vi "svx_Shortcut Menu.vi"(7 "waveform graph?":bool, 9 "Container State":T3, 10 "Display State In":T1={"X Scale Width %"=50.0, "Y Scale Height %"=50.0, "X-Axis Range"={"Minimum"=0.0, "Maximum"=10.0}, "Y-Axis Range"={"Minimum"=0.0, "Maximum"=10.0}, "Z-Axis Range"={"Minimum"=0.0, "Maximum"=10.0}, "Plot Color"=61212, "Frame Color"=16252785, "Background Color"=16777222, "Initial AutoScale Y"=TRUE, "AutoScale X"=2, "AutoScale Y"=2, "AutoScale Z"=2, "Plot Transparency"=FALSE, "X-Axis Name"="Frequency", "Y-Axis Name"="Amplitude", "Z-Axis Name"="", "X-Axis Scaling Factor"={"Offset"=0.0, "Multiplier"=1.0}, "Y-Axis Scaling Factor"={"Offset"=0.0, "Multiplier"=1.0}, "Z-Axis Scaling Factor"={"Offset"=0.0, "Multiplier"=1.0}, "X-Scale Visible"=TRUE, "Y-Scale Visible"=TRUE, "Z-Scale Visible"=TRUE, "X-Scale Label Visible"=TRUE, "Y-Scale Label Visible"=TRUE, "Z-Scale Label Visible"=TRUE, "X-Axis Range Scaled"={"Minimum"=0.0, "Maximum"=10.0}, "Y-Axis Range Scaled"={"Minimum"=0.0, "Maximum"=10.0}, "Z-Axis Range Scaled"={"Minimum"=0.0, "Maximum"=10.0}, "Rev Z Order"=FALSE, "X-Scale Format Str"="%#.4g", "Y-Scale Format Str"="%#.4g", "Z-Scale Format Str"="%#.4g", "Decor color"=12369084, "Scale Range Change"=refnum, "out of state queue"=refnum, "property nodes"=refnum, "Lines"=[], "Line Properties"={"Line Color"=61212, "Line Width"=61212, "Line Style"=enum."Dash", "DisplayLines"=FALSE}} {"Line Properties"."Line Width" min=1}, 11 "menu reference in":refnum<k9>) -> (3 "menu referenceout":refnum<k9>)   [LabVIEW 2017, in "SVX Waterfall Graph.xctl"]
uses:
  <vilib>/addons/_XControls/Waterfall Graph/SVX Waterfall Graph.xctl
  <vilib>/_xctls/Container State.ctl
  <vilib>/addons/_XControls/Waterfall Graph/subVIs/svx_Waterfall State.ctl
  <vilib>/addons/_NISVFA/_Shared subVIs/Controls/svc_Cluster of Array of Cluster of XYZ.ctl
  <vilib>/_xctls/XControlSupport.lvlib
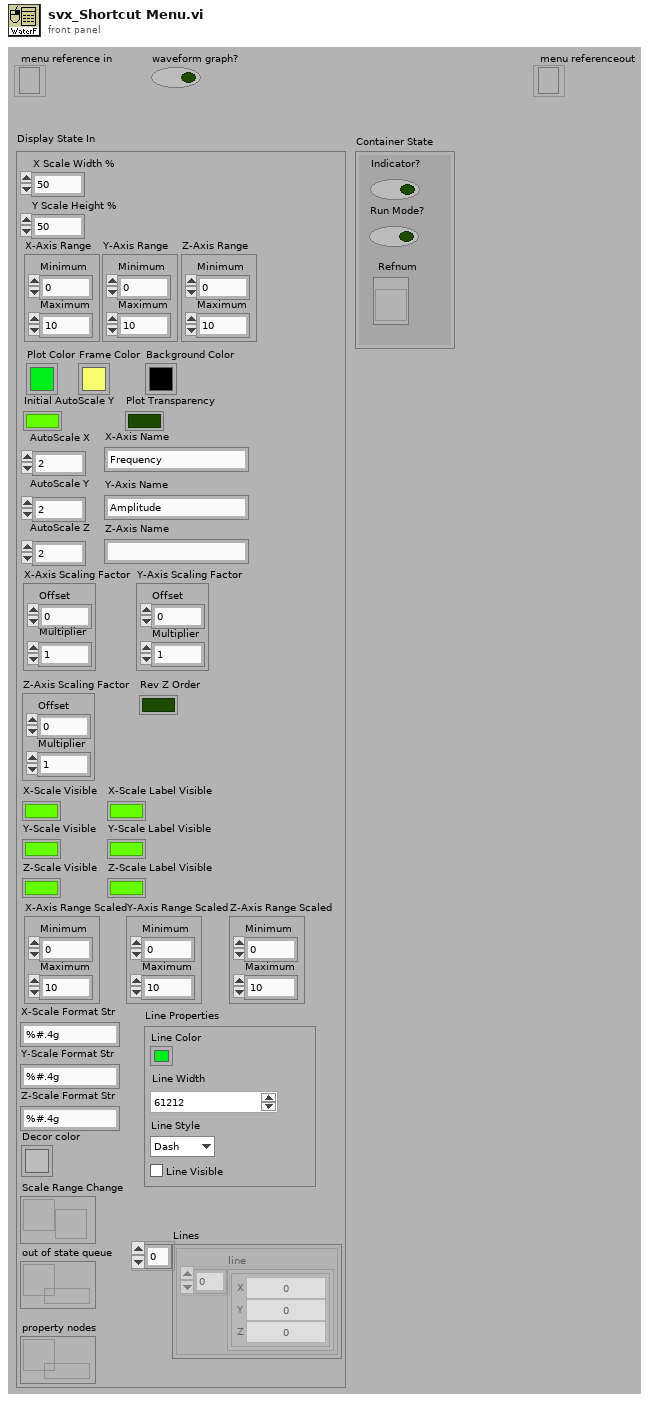
[diagram p1: front panel]
types:
  T1 = typedef "SVX Waterfall Graph.xctl/svx_Waterfall State.ctl" = cluster{"X Scale Width %":dbl, "Y Scale Height %":dbl, "X-Axis Range":cluster{"Minimum":dbl, "Maximum":dbl}, "Y-Axis Range":cluster{"Minimum":dbl, "Maximum":dbl}, "Z-Axis Range":cluster{"Minimum":dbl, "Maximum":dbl}, "Plot Color":u32, "Frame Color":u32, "Background Color":u32, "Initial AutoScale Y":bool, "AutoScale X":u8, "AutoScale Y":u8, "AutoScale Z":u8, "Plot Transparency":bool, "X-Axis Name":string, "Y-Axis Name":string, "Z-Axis Name":string, "X-Axis Scaling Factor":cluster{"Offset":dbl, "Multiplier":dbl}, "Y-Axis Scaling Factor":cluster{"Offset":dbl, "Multiplier":dbl}, "Z-Axis Scaling Factor":cluster{"Offset":dbl, "Multiplier":dbl}, "X-Scale Visible":bool, "Y-Scale Visible":bool, "Z-Scale Visible":bool, "X-Scale Label Visible":bool, "Y-Scale Label Visible":bool, "Z-Scale Label Visible":bool, "X-Axis Range Scaled":cluster{"Minimum":dbl, "Maximum":dbl}, "Y-Axis Range Scaled":cluster{"Minimum":dbl, "Maximum":dbl}, "Z-Axis Range Scaled":cluster{"Minimum":dbl, "Maximum":dbl}, "Rev Z Order":bool, "X-Scale Format Str":string, "Y-Scale Format Str":string, "Z-Scale Format Str":string, "Decor color":u32, "Scale Range Change":refnum<user-event>, "out of state queue":refnum<queue>, "property nodes":refnum<queue>, "Lines":T2[], "Line Properties":cluster{"Line Color":u32, "Line Width":u16, "Line Style":enum32{"Solid", "Dash", "Dot", "DashDot", "DashDotDot"}, "DisplayLines":bool}}
  T2 = typedef "svc_Cluster of Array of Cluster of XYZ.ctl" = cluster{"line":cluster{"X":dbl, "Y":dbl, "Z":dbl}[]}
  T3 = typedef "XControlSupport.lvlib/Container State.ctl" = cluster{"Indicator?":bool, "Run Mode?":bool, " Refnum":refnum<vi>}
  T4 = cluster{"menu tag":string, "items to delete":string[], "new menu":cluster{"item names":string, "item tags":string, "after item":string}[], "root?":bool}
  T5 = cluster{"menu tag":string, "items to delete":string[], "new menu":cluster{"item names":string, "item tags":string, "after item":string}[], "root?":bool}[]
  T6 = cluster{"item names":string, "item tags":string, "after item":string}[]
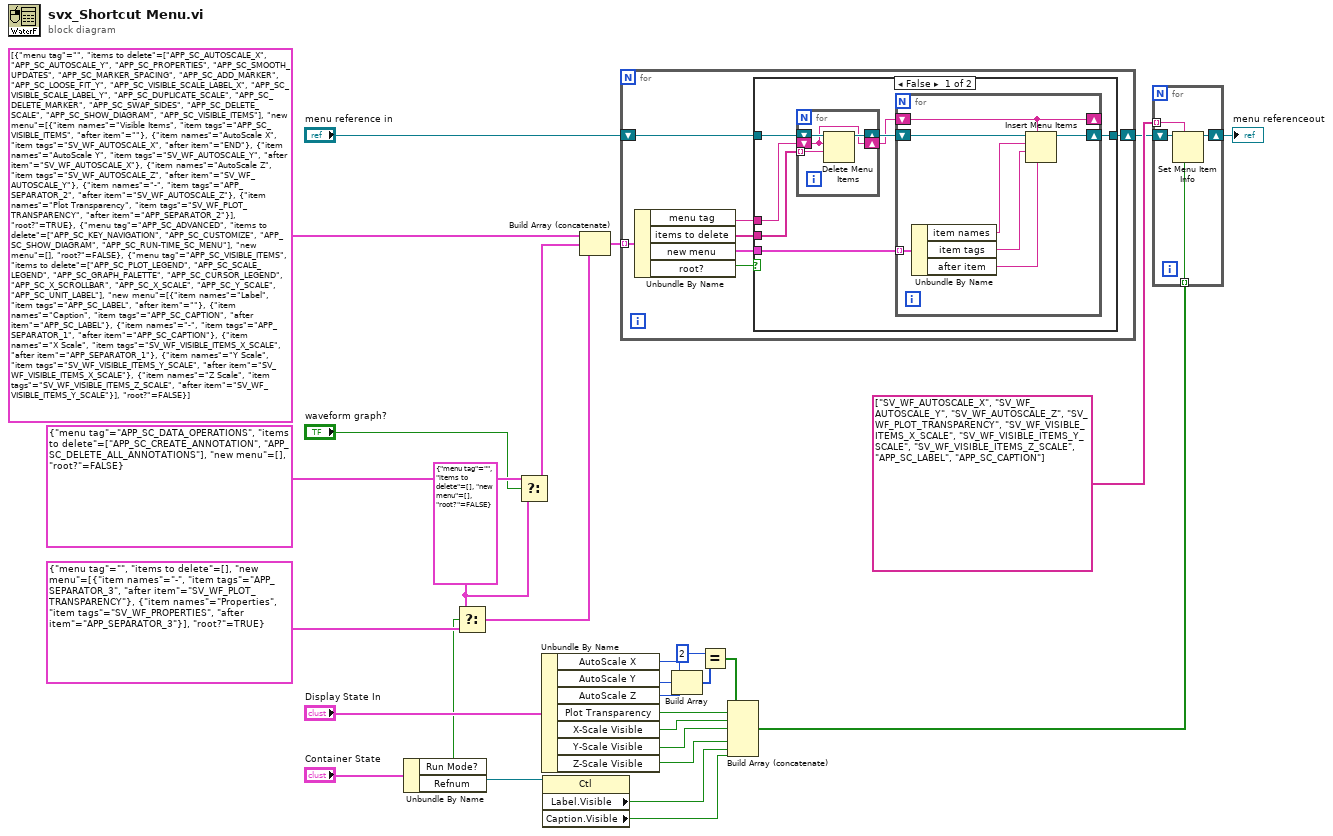
[diagram p0: block diagram]
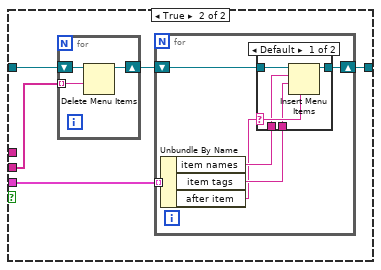
[diagram p2: hidden frame]
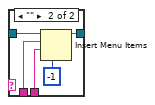
[diagram p3: hidden frame]
diagram:
  w26 = T4 {"menu tag"="", "items to delete"=[], "new menu"=[], "root?"=FALSE} ("t")
  n1 = Unbundle By Name("Container State") -> ("Run Mode?"=w2:bool, "Refnum"=w19:refnum<vi>)
  n2 = Select(t=w26, s=w2, f=T4 {"menu tag"="", "items to delete"=[], "new menu"=[{"item names"="-", "item tags"="APP_SEPARATOR_3", "after item"="SV_WF_PLOT_TRANSPARENCY"}, {"item names"="Properties", "item tags"="SV_WF_PROPERTIES", "after item"="APP_SEPARATOR_3"}], "root?"=TRUE} ("menu item")) -> (s? t:f=w23:T4)
  n3 = Select(t=T4 {"menu tag"="APP_SC_DATA_OPERATIONS", "items to delete"=["APP_SC_CREATE_ANNOTATION", "APP_SC_DELETE_ALL_ANNOTATIONS"], "new menu"=[], "root?"=FALSE} ("menu item"), s="waveform graph?", f=w26) -> (s? t:f=w24:T4)
  n4 = Unbundle By Name("Display State In") -> ("AutoScale X"=w14:u8, "AutoScale Y"=w15:u8, "AutoScale Z"=w12:u8, "Plot Transparency"=w11:bool, "X-Scale Visible"=w16:bool, "Y-Scale Visible"=w17:bool, "Z-Scale Visible"=w18:bool)
  n5 = property class="Ctl"(reference=w19) -> ("Label.Visible"=w20:bool, "Caption.Visible"=w21:bool)  [unwired: 1 in, 2 out]
  n6 = Build Array (concatenate)(T5 [{"menu tag"="", "items to delete"=["APP_SC_AUTOSCALE_X", "APP_SC_AUTOSCALE_Y", "APP_SC_PROPERTIES", "APP_SC_SMOOTH_UPDATES", "APP_SC_MARKER_SPACING", "APP_SC_ADD_MARKER", "APP_SC_LOOSE_FIT_Y", "APP_SC_VISIBLE_SCALE_LABEL_X", "APP_SC_VISIBLE_SCALE_LABEL_Y", "APP_SC_DUPLICATE_SCALE", "APP_SC_DELETE_MARKER", "APP_SC_SWAP_SIDES", "APP_SC_DELETE_SCALE", "APP_SC_SHOW_DIAGRAM", "APP_SC_VISIBLE_ITEMS"], "new menu"=[{"item names"="Visible Items", "item tags"="APP_SC_VISIBLE_ITEMS", "after item"=""}, {"item names"="AutoScale X", "item tags"="SV_WF_AUTOSCALE_X", "after item"="END"}, {"item names"="AutoScale Y", "item tags"="SV_WF_AUTOSCALE_Y", "after item"="SV_WF_AUTOSCALE_X"}, {"item names"="AutoScale Z", "item tags"="SV_WF_AUTOSCALE_Z", "after item"="SV_WF_AUTOSCALE_Y"}, {"item names"="-", "item tags"="APP_SEPARATOR_2", "after item"="SV_WF_AUTOSCALE_Z"}, {"item names"="Plot Transparency", "item tags"="SV_WF_PLOT_TRANSPARENCY", "after item"="APP_SEPARATOR_2"}], "root?"=TRUE}, {"menu tag"="APP_SC_ADVANCED", "items to delete"=["APP_SC_KEY_NAVIGATION", "APP_SC_CUSTOMIZE", "APP_SC_SHOW_DIAGRAM", "APP_SC_RUN-TIME_SC_MENU"], "new menu"=[], "root?"=FALSE}, {"menu tag"="APP_SC_VISIBLE_ITEMS", "items to delete"=["APP_SC_PLOT_LEGEND", "APP_SC_SCALE_LEGEND", "APP_SC_GRAPH_PALETTE", "APP_SC_CURSOR_LEGEND", "APP_SC_X_SCROLLBAR", "APP_SC_X_SCALE", "APP_SC_Y_SCALE", "APP_SC_UNIT_LABEL"], "new menu"=[{"item names"="Label", "item tags"="APP_SC_LABEL", "after item"=""}, {"item names"="Caption", "item tags"="APP_SC_CAPTION", "after item"="APP_SC_LABEL"}, {"item names"="-", "item tags"="APP_SEPARATOR_1", "after item"="APP_SC_CAPTION"}, {"item names"="X Scale", "item tags"="SV_WF_VISIBLE_ITEMS_X_SCALE", "after item"="APP_SEPARATOR_1"}, {"item names"="Y Scale", "item tags"="SV_WF_VISIBLE_ITEMS_Y_SCALE", "after item"="SV_WF_VISIBLE_ITEMS_X_SCALE"}, {"item names"="Z Scale", "item tags"="SV_WF_VISIBLE_ITEMS_Z_SCALE", "after item"="SV_WF_VISIBLE_ITEMS_Y_SCALE"}], "root?"=FALSE}] ("edit-time menu"), w24, w23) -> (w22:T5)
  n7 = for {
    tunnel: w22 -> [w36] mode=indexing
    shift-right: [w31] -> w5
    shift-left: "menu reference in" -> [w35]
    n8 = Unbundle By Name(w36) -> ("menu tag"=w34:string, "items to delete"=w33:string[], "new menu"=w32:T6, "root?"=w30:bool)
    n9 = case shown="False" w30 {
      tunnel: w35 -> [w43 w59]
      tunnel: w34 -> [w42 _]
      tunnel: w33 -> [w41 w58]
      tunnel: w32 -> [w38 w56]
      tunnel: [w37 w55] -> w31
      frame False {
        n10 = for {
          shift-right: [w53] -> w40
          shift-left: w43 -> [w54]
          shift-right: [w51] -> w39
          shift-left: w42 -> [w51]
          tunnel: w41 -> [w52] mode=indexing
          n11 = Delete Menu Items(7:w52, 8:w51, 9:w54) -> (3:w53:refnum<k9>)  [unwired: 1 in, 1 out]
        }
        n12 = for {
          shift-right: [w44] -> w37
          shift-left: w40 -> [w50]
          shift-right: [w49] -> _
          shift-left: w39 -> [w49]
          tunnel: w38 -> [w48] mode=indexing
          n13 = Unbundle By Name(w48) -> ("item names"=w47:string, "item tags"=w46:string, "after item"=w45:string)
          n14 = Insert Menu Items(4:w45, 5:w49, 7:w46, 8:w47, 9:w50) -> (3:w44:refnum<k9>)  [unwired: 1 in, 2 out]
        }
      }
      frame True {
        n15 = for {
          shift-right: [w77] -> w57
          shift-left: w59 -> [w78]
          tunnel: w58 -> [w76] mode=indexing
          n16 = Delete Menu Items(7:w76, 9:w78) -> (3:w77:refnum<k9>)  [unwired: 2 in, 1 out]
        }
        n17 = for {
          shift-right: [w65] -> w55
          shift-left: w57 -> [w64]
          tunnel: w56 -> [w63] mode=indexing
          n18 = Unbundle By Name(w63) -> ("item names"=w62:string, "item tags"=w61:string, "after item"=w60:string)
          n19 = case shown="Default" w60 {
            selector: w60 -> [w68 _]
            tunnel: [w69 w75] -> w65
            tunnel: w64 -> [w70 w74]
            tunnel: w62 -> [w67 w73]
            tunnel: w61 -> [w66 w72]
            frame Default {
              n20 = Insert Menu Items(4:w68, 7:w66, 8:w67, 9:w70) -> (3:w69:refnum<k9>)  [unwired: 2 in, 2 out]
            }
            frame "" {
              n21 = Insert Menu Items(4:-1, 7:w72, 8:w73, 9:w74) -> (3:w75:refnum<k9>)  [unwired: 2 in, 2 out]
            }
          }
        }
      }
    }
  }
  n22 = Build Array(w14, w15, w12) -> (w13:u8[])
  n23 = Equal?(x=u8 2 ("y"), y=w13) -> (x = y?=w10:bool[])
  n24 = Build Array (concatenate)(w10, w11, w16, w17, w18, w20, w21) -> (w4:bool[])
  n25 = for {
    tunnel: string[] ["SV_WF_AUTOSCALE_X", "SV_WF_AUTOSCALE_Y", "SV_WF_AUTOSCALE_Z", "SV_WF_PLOT_TRANSPARENCY", "SV_WF_VISIBLE_ITEMS_X_SCALE", "SV_WF_VISIBLE_ITEMS_Y_SCALE", "SV_WF_VISIBLE_ITEMS_Z_SCALE", "APP_SC_LABEL", "APP_SC_CAPTION"] -> [w82] mode=indexing
    tunnel: w4 -> [w80] mode=indexing
    shift-right: [w79] -> w3
    shift-left: w5 -> [w81]
    n26 = Set Menu Item Info(6:w80, 7:w82, 11:w81) -> (3:w79:refnum<k9>)  [unwired: 4 in, 1 out]
  }
  "menu referenceout" <- w3
